vi "LV86_Divide.vi"(0 "Constant":dbl=1.0, 2 "Image 2":T1={"Width"=0, "Height"=0, "Depth"=-1, "data"=[], "Compressed data"=[], "Color table"=[], "Duration"=0, "Options"=0, "Timestamp"=0, "ID"=0, "Reserved"=0, "Dialogs"=0} {"Dialogs" format="%.0b"}, 3 "Image":T1 {"Dialogs" format="%.0b"}) -> (1 "Image Out":T1 {"Dialogs" format="%.0b"})   [LabVIEW 2024]
doc: "This VI divides two images pixel by pixel or divides an image by a constant. If <B>Image 2</B> is unwired, the image is divided by the <B>constant</B>. (Does not work on a color image)"
uses:
  <userlib>/ImageProcessing/QTLIB_2595_LV86/QT_Image.ctl
panel:
  # "This VI divides two images pixel by pixel or a constant\n to one image.  If Image 2 is unwired, the constant \nis divided into the image. (Does not work on a color image)"
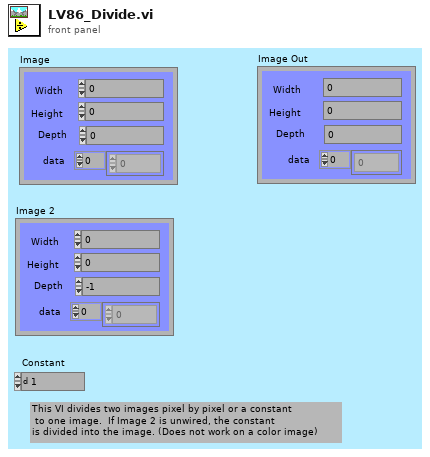
[diagram p1: front panel]
types:
  T1 = typedef "QT_Image.ctl" = cluster{"Width":i32, "Height":i32, "Depth":i32, "data":u8[], "Compressed data":u8[], "Color table":u32[], "Duration":i32, "Options":i32, "Timestamp":i32, "ID":i32, "Reserved":i32, "Dialogs":u32}
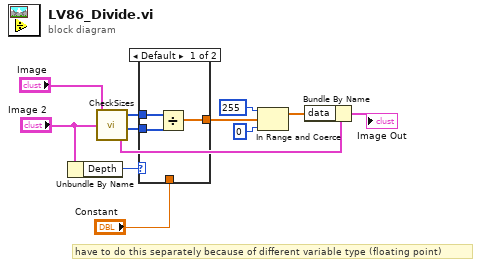
[diagram p0: block diagram]
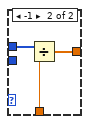
[diagram p2: hidden frame]
diagram:
  # "have to do this separately because of different variable type (floating point)"
  n1 = Unbundle By Name("Image 2") -> ("Depth"=w3:i32)
  n2 = call <userlib>:"CheckSizes.vi"("Image 2"="Image 2", "Image"="Image") -> ("Image template"=w5:T1, "Image 2 data"=w1:u8[], "Image 1 data"=w6:i32[])  [unwired: 1 in]
  n3 = case shown="Default" w3 {
    tunnel: [w14 w18] -> w9
    tunnel: w6 -> [w15 w17]
    tunnel: "Constant" -> [_ w16]
    tunnel: w1 -> [w13 _]
    frame Default {
      n4 = Divide(x=w15, y=w13) -> (x/y=w14:dbl[])
    }
    frame -1 {
      n5 = Divide(x=w17, y=w16) -> (x/y=w18:dbl[])
    }
  }
  n6 = In Range and Coerce(upper limit=u8 255, x=w9, lower limit=u8 0) -> (coerced(x)=w12:dbl[])  [unwired: 1 out]
  n7 = Bundle By Name(cluster=w5, "data"=w12) -> (→"Image Out":T1)
